vi "RSZVB Get Marker State.vi"(8 "error in (no error)":errorcluster {"code" format="%.0x"}, 9 "Marker (1)":i32=1, 10 "Channel (Trace) (1)":i32=1, 11 "VISA session":refnum<visa-resource-name>) -> (0 "error out":errorcluster {"code" format="%.0x"}, 2 "Marker State":bool, 3 "dup VISA session":refnum<visa-resource-name>)   [LabVIEW 2011]
doc: "This VI returns if the marker numbered <Mk> is assigned to trace no. <Ch/Tr>.\n\nRemote-control command(s):\nCALCulate<Ch/Tr>:MARKer<Mk>[:STATe]?"
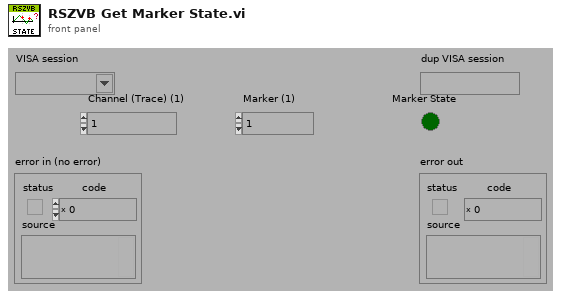
[diagram p1: front panel]
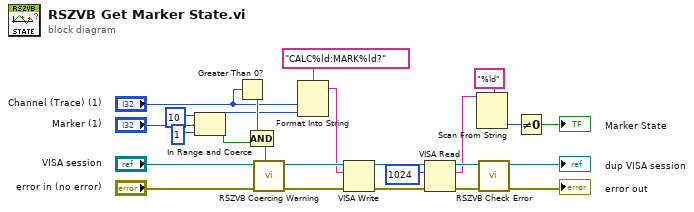
[diagram p0: block diagram]
diagram:
  n1 = In Range and Coerce(upper limit=10, x="Marker (1)", lower limit=1) -> (coerced(x)=w7:i32, In Range?=w8:bool)
  n2 = Greater Than 0?(x="Channel (Trace) (1)") -> (x > 0?=w11:bool)
  n3 = Compound Arithmetic op=AND(w11, w8) -> (w13:bool)
  n4 = call "RSZVB Coercing Warning.vi"("In Range?"=w13, "error in (no error)"="error in (no error)", "VISA session"="VISA session") -> ("error out"=w14:errorcluster, "dup VISA session"=w15:refnum<visa-resource-name>)  [unwired: 7 in]
  n5 = Format Into String(format string="CALC%ld:MARK%ld?", "Channel (Trace) (1)", w7) -> (resulting string=w12:string)  [unwired: 2 in, 1 out]
  n6 = VISA Write(VISA resource name=w15, write buffer=w12, error in (no error)=w14) -> (VISA resource name out=w5:refnum<visa-resource-name>, error out=w6:errorcluster)  [unwired: 1 out]
  n7 = VISA Read(VISA resource name=w5, byte count=u32 1024 ("byte count (0)"), error in (no error)=w6) -> (VISA resource name out=w24:refnum<visa-resource-name>, read buffer=w21:string, error out=w23:errorcluster)  [unwired: 1 out]
  n8 = Scan From String(format string="%ld", input string=w21) -> (output 1=w20:i32)  [unwired: 3 in, 3 out]
  n9 = call "RSZVB Check Error.vi"("error in (no error)"=w23, "VISA session"=w24) -> ("error out"=→"error out":errorcluster, "dup VISA session"=→"dup VISA session":refnum<visa-resource-name>)  [unwired: 8 in]
  n10 = Not Equal To 0?(x=w20) -> (x != 0?=→"Marker State":bool)
